vi "ROI entry screen-Analyse ROI lengths.vi"(11 "Old ROI file's data in":dbl[][](array[numeric])) -> (0 "Lines-Equal to the first value?":bool[](array[boolean]), 1 "Number of lines []":dbl[](array[numeric]), 2 "Lengths-Equal to the first value?":bool[](array[boolean]), 3 "Length []":dbl[](array[numeric]), 4 "Vertical?":bool[](array[boolean]))   [LabVIEW 2013]
panel:
  # "The length is always the longest dimension"
  # "The number of lines is always the shortest dimension"
  # "RE-ENTRANT"
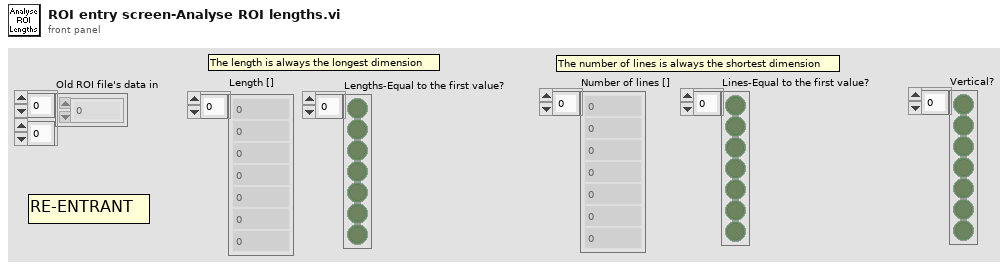
[diagram p1: front panel]
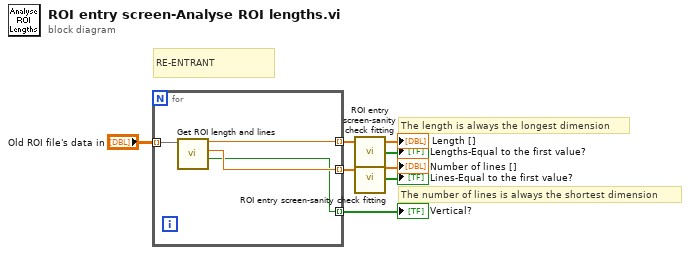
[diagram p0: block diagram]
diagram:
  # "The number of lines is always the shortest dimension"
  # "The length is always the longest dimension"
  # "RE-ENTRANT"
  n1 = for {
    tunnel: "Old ROI file's data in" -> [w12] mode=indexing
    tunnel: [w11] -> w4 mode=indexing
    tunnel: [w10] -> w3 mode=indexing
    tunnel: [w9] -> w1 mode=indexing
    n2 = call "Get ROI length and lines.vi"("Old ROI file's data in"=w12) -> ("Vertical"=w9:bool, "Number of lines"=w10:dbl, "Length"=w11:dbl)  [unwired: 8 in]
  }
  "Vertical?" <- w1
  n3 = call "ROI entry screen-sanity check fitting.vi"("Array in"=w4) -> ("Equal to the first value?"=→"Lengths-Equal to the first value?":bool[], "Array out"=→"Length []":dbl[])  [unwired: 3 in]
  n4 = call "ROI entry screen-sanity check fitting.vi"("Array in"=w3) -> ("Equal to the first value?"=→"Lines-Equal to the first value?":bool[], "Array out"=→"Number of lines []":dbl[])  [unwired: 3 in]
